vi "bulk read.vi"(7 "timeout":i32, 9 "size":i32, 11 "ep":i32) -> (3 "len":i32)   [LabVIEW 2013, in "libusvlv.lvlib"]
doc: "extern \"C\" int _declspec_dll_use bulk_read(int ep, char* bytes, int size, int timeout);"
uses:
  libusvlv.lvlib
  UsbCom.dll
panel:
  in  "element":i8
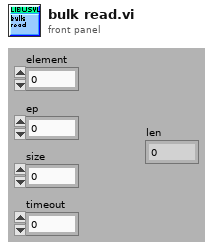
[diagram p1: front panel]
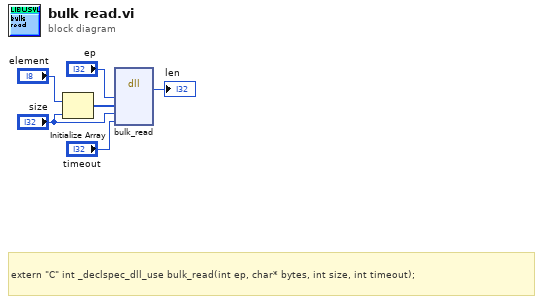
[diagram p0: block diagram]
diagram:
  # "extern \"C\" int _declspec_dll_use bulk_read(int ep, char* bytes, int size, int timeout);"
  n1 = Initialize Array("element", "size") -> (w3:i8[])
  n2 = dll-call lib="E:/libusvlv/UsbCom.dll" fn="bulk_read"("ep"="ep", "bytes"=w3, "size"="size", "timeout"="timeout") -> ("返回类型"=→"len":i32)  [unwired: 7 in, 2 out]
